vi "Get Lockin Result.vi"(5 "Result in":refnum<class "Acquired Result.lvclass">, 6 "Init work":bool, 7 "Update period":dbl, 8 "error in (no error)":errorcluster, 9 "Last request":bool, 10 "Requester":string, 11 "Red Pitaya Digitizer in":refnum<class "Red Pitaya Digitizer.lvclass">) -> (0 "error out":errorcluster, 1 "Valid result":bool, 2 "Result out":refnum<class "Acquired Result.lvclass">, 3 "Red Pitaya Digitizer out":refnum<class "Red Pitaya Digitizer.lvclass">)   [LabVIEW 2024, in "Red Pitaya Digitizer.lvclass"]
uses:
  Red Pitaya Digitizer.lvclass
  Instruments/Results/Acquired Result/Acquired Result.lvclass
  <vilib>/Utility/error.llb/Error Cluster From Error Code.vi
  RP Core/RP Instrument/RP Instrument.lvclass
  <vilib>/ErrorRing/Error Ring.xnode
  Instruments/Pulse Driver/Lockin Digitizer Driver/Lockin Digitizer Driver.lvclass
  Red Pitaya Digitizer.lvclass/Red Pitaya Digitizer.ctl
  File/File Class/File.lvclass
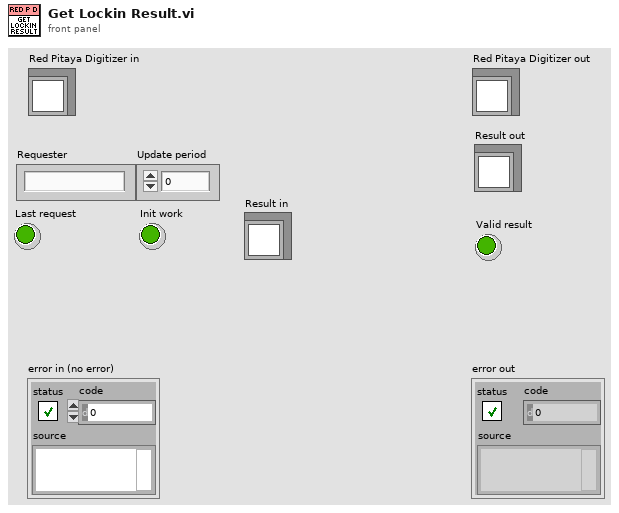
[diagram p1: front panel]
types:
  T1 = typedef "Lockin Digitizer Configuration.ctl" = cluster{"Post-trigger delay":dbl, "Post-trigger duration":dbl, "Rate":dbl, "Ranges":dbl[], "Re-name channels":string[], "Active channels":string, "External\nclock":bool, "Monitor time\nconstant":dbl, "Sync":bool, "Lock-in input channel phases":dbl[], "Output channels configuration":T2[]}
  T2 = typedef "Output Channel Configuration.ctl" = cluster{"Input channels":string, "Frequency":dbl, "Output amplitude":dbl, "Output channel number":i32}
  T3 = map{i32, cluster{"Module":i32, "Local channel":i32}}
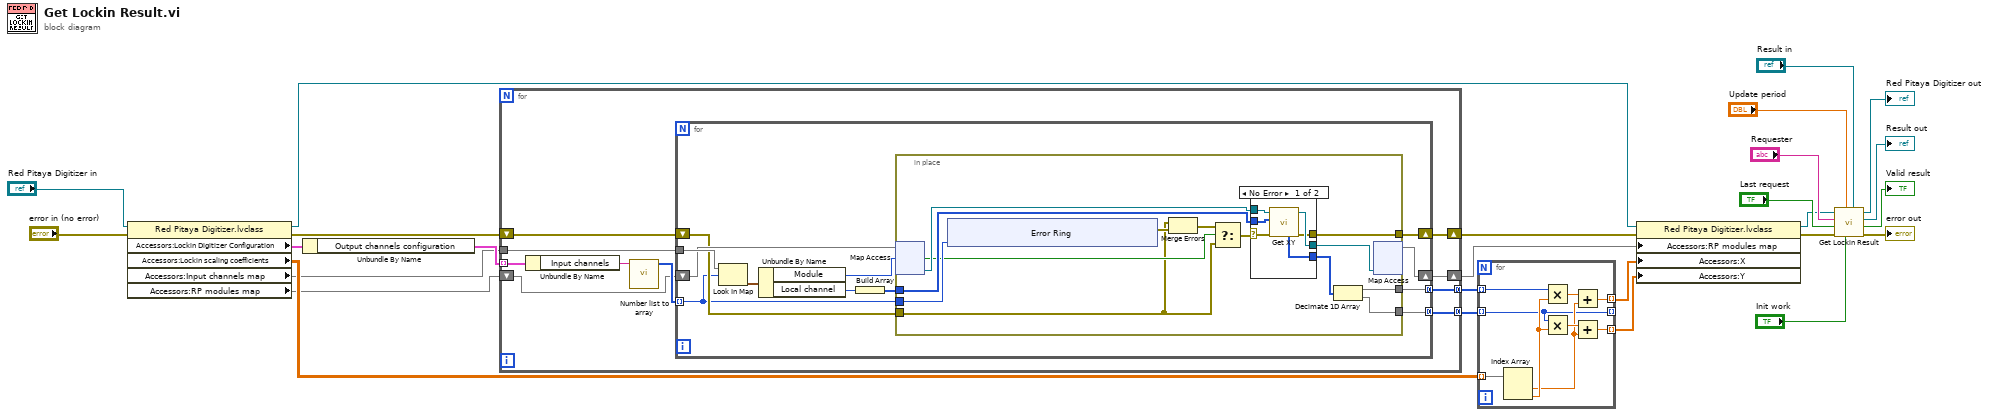
[diagram p0: block diagram]
diagram:
  n1 = property class="Red Pitaya Digitizer.lvclass"(reference="Red Pitaya Digitizer in", error in="error in (no error)") -> (reference out=w12:refnum<class "Red Pitaya Digitizer.lvclass">, error out=w5:errorcluster, "Accessors:Lockin Digitizer Configuration"=w16:T1, "Accessors:Lockin scaling coefficients"=w10:dbl[][], "Accessors:Input channels map"=w7:T3, "Accessors:RP modules map "=w6:map{i32, refnum<class "RP Instrument.lvclass">})
  n2 = Unbundle By Name(w16) -> ("Output channels configuration"=w8:T2[])
  n3 = for {
    tunnel: w8 -> [w36] mode=indexing
    tunnel: w7 -> [w33]
    shift-right: [w27] -> w2
    shift-left: w6 -> [w32]
    shift-right: [w30] -> w1
    shift-left: w5 -> [w31]
    tunnel: [w29] -> w4 mode=concatenating
    tunnel: [w28] -> w3 mode=concatenating
    n4 = Unbundle By Name(w36) -> ("Input channels"=w35:string)
    n5 = call "Number list to array.vi"("Number list"=w35) -> ("Number list array"=w34:i32[])  [unwired: 7 in, 3 out]
    n6 = for {
      tunnel: w34 -> [w37] mode=indexing
      tunnel: w33 -> [w48]
      shift-right: [w38] -> w27
      shift-left: w32 -> [w45]
      shift-right: [w41] -> w30
      shift-left: w31 -> [w42]
      tunnel: [w40] -> w29 mode=concatenating
      tunnel: [w39] -> w28 mode=concatenating
      n7 = Look In Map(map=w48, key=w37) -> (value=w47:cluster{"Module":i32, "Local channel":i32})  [unwired: 1 in, 1 out]
      n8 = Unbundle By Name(w47) -> ("Module"=w44:i32, "Local channel"=w46:i32)
      n9 = Build Array(w46) -> (w43:i32[])
      n10 = in-place {
        in-place-border: w43 -> [w61]
        in-place-border: w42 -> [w50]
        in-place-border: [w58] -> w41
        in-place-border: [w56] -> w40
        in-place-border: [w55] -> w39
        in-place-border: w37 -> [w52]
        n11 = in-place-map #1(w45, w44) -> (w60:refnum<class "RP Instrument.lvclass">, w51:bool)  [unwired: 1 in]
        n12 = xnode "Error Ring"("parameter 0"=w52) -> ("error out"=w54:errorcluster)
        n13 = Merge Errors(w50, w54) -> (w53:errorcluster)
        n14 = Select(t=w53, s=w51, f=w50) -> (s? t:f=w49:errorcluster)
        n15 = case shown="No Error" w49 {
          selector: w49 -> [w62 w68]
          tunnel: w61 -> [w67 _]
          tunnel: w60 -> [w66 w69]
          tunnel: [w65 w69] -> w59
          tunnel: [w64 w68] -> w58
          tunnel: [w63 _] -> w57
          frame No Error {
            n16 = call-dynamic "Get XY.vi"("error in (no error)"=w62, "Channels"=w67, "RP Instrument in"=w66) -> ("error out"=w64:errorcluster, "RP Instrument out"=w65:refnum<class "RP Instrument.lvclass">, "Signal"=w63:i32[])  [unwired: 6 in]
          }
          frame Error {
          }
        }
        n17 = Decimate 1D Array(w57) -> (w56:i32[], w55:i32[])
        n18 = in-place-map #1(w59) -> (w38:map{i32, refnum<class "RP Instrument.lvclass">})  [unwired: 1 in, 2 out]
      }
    }
  }
  n19 = for {
    tunnel: w10 -> [w85] mode=indexing
    tunnel: [w83] -> w11 mode=indexing
    tunnel: [w77] -> _ mode=indexing
    tunnel: [w79] -> w9 mode=indexing
    tunnel: w4 -> [w78] mode=indexing
    tunnel: w3 -> [w77] mode=indexing
    n20 = Index Array(array=w85) -> (element #1=w80:dbl, element #2=w82:dbl)  [unwired: 2 in]
    n21 = Multiply(x=w78, y=w82) -> (x*y=w81:dbl)
    n22 = Multiply(x=w77, y=w82) -> (x*y=w84:dbl)
    n23 = Add(x=w81, y=w80) -> (x+y=w79:dbl)
    n24 = Add(x=w84, y=w80) -> (x+y=w83:dbl)
  }
  n25 = property class="Red Pitaya Digitizer.lvclass"(reference=w12, error in=w1, "Accessors:RP modules map "=w2, "Accessors:X"=w9, "Accessors:Y"=w11) -> (reference out=w15:refnum<class "Red Pitaya Digitizer.lvclass">, error out=w13:errorcluster)
  n26 = call-parent "Get Lockin Result.vi"("Result in"="Result in", "Init work"="Init work", "Update period"="Update period", "error in (no error)"=w13, "Last request"="Last request", "Requester"="Requester", "Lockin Digitizer Driver in"=w15) -> ("error out"=→"error out":errorcluster, "Valid result"=→"Valid result":bool, "Result out"=→"Result out":refnum<class "Acquired Result.lvclass">, "Lockin Digitizer Driver out"=→"Red Pitaya Digitizer out":refnum<class "Red Pitaya Digitizer.lvclass">)  [unwired: 1 in]
